vi "MacroGen_MD_old.vi"() -> ()   [LabVIEW 2012]
uses:
  Custom Controls and Typedefs/Available Operations Tree.ctl
  Custom Controls and Typedefs/Edit Button.ctl
  Custom Controls and Typedefs/Delete Button.ctl
  Custom Controls and Typedefs/Macro_MD_UI Control Refnums.ctl
  SubVIs/FormatTree&TableStyle_Commands.ctl
  SubVIs/FGV_MacroGen_Commands.ctl
  Custom Controls and Typedefs/Macro_CommandStruct.ctl
  Custom Controls and Typedefs/Macro_Action_List.ctl
  Custom Controls and Typedefs/Macro_ArgumentStruct.ctl
  CommonResource VIs/FormatTableStyle_Commands.ctl
  <vilib>/Utility/file.llb/Write To Spreadsheet File (string).vi
panel:
  in  "MacroTreeOperation":T3
  in  "File Operation Cluster":cluster{"Load Macro":bool, "SaveAs":bool}
  in  "Table Navigation Cluster":T4
  in  "Parameters":string[][](table)
  in  "Execute Macro":bool
  in  "Add":bool
  in  "Available Actions":T5
  in  "stop":bool
  in  "Macro":string(tree)
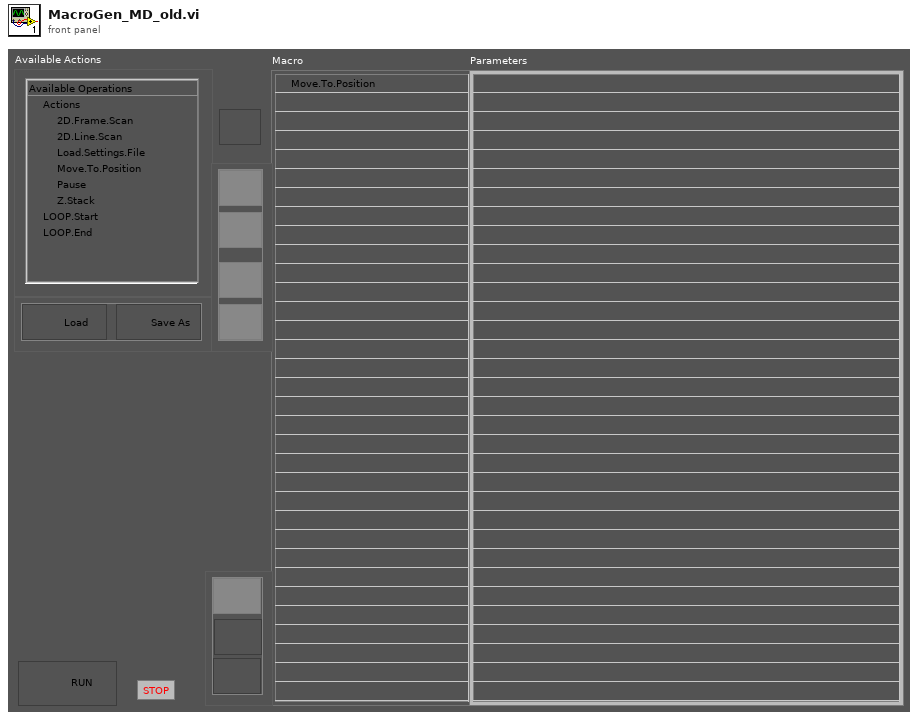
[diagram p1: front panel]
types:
  T1 = typedef "Edit Button.ctl" = bool
  T2 = typedef "Delete Button.ctl" = bool
  T3 = cluster{"Save Button":bool, "Edit Button":T1, "Delete Button":T2}
  T4 = cluster{"Table Index Up":bool, "Table Index Up-End":bool, "Table Index Down":bool, "Table Index Down-End":bool}
  T5 = typedef "Available Operations Tree.ctl" = string
  T6 = typedef "Macro_MD_UI Control Refnums.ctl" = cluster{"Available Operations":refnum<vi>, "Created Macro":refnum<vi>, "Indent Item":refnum<vi>, "Add Selected to Macro":refnum<vi>, "Outdent Item":refnum<vi>, "Number of Iterations":refnum<vi>, "Seconds to Wait":refnum<vi>, "Load Macro":refnum<vi>, "Save Macro":refnum<vi>, "Select File to Load":refnum<vi>, "Params Table":refnum<vi>, "Delete":refnum<vi>, "Edit Button":refnum<vi>, "Execute Macro":refnum<vi>}
  T7 = typedef "FGV_MacroGen_Commands.ctl" = enum16{"Initialize", "Get Array", "Load from file", "Insert Item", "Insert at End", "Edit Item", "Delete Item", "Move Items", "Save", "SaveAs"}
  T8 = typedef "FormatTree&TableStyle_Commands.ctl" = enum16{"Colour Row", "Uncolour Row", "Bold Row", "Unbold Row", "Clear", "UpdateVisibleRows"}
  T9 = typedef "Macro_CommandStruct.ctl" = cluster{"Action":T10, "Arguments":T11[]}
  T10 = typedef "Macro_Action_List.ctl" = enum16{"Unknown", "2D.Frame.Scan", "2D.Line.Scan", "Load.Settings.File", "Move.To.Position", "Pause", "Z.Stack", "LOOP.Start", "LOOP.End"}
  T11 = typedef "Macro_ArgumentStruct.ctl" = cluster{"ArgumentName":string, "DataType":enum16{"Numeric", "String"}, "Value":variant}
  T12 = typedef "FormatTableStyle_Commands.ctl" = enum16{"Colour Row", "Uncolour Row", "Bold Row", "Clear table", "UpdateVisibleRows"}
  T13 = cluster{"data name":string, "drag data":variant}[]
  T14 = typedef "LVPoint32TypeDef.ctl" = cluster{"Horizontal":i32, "Vertical":i32}
  T15 = typedef "LVRowAndColumnTypeDef.ctl" = cluster{"Row":i32, "Column":i32}
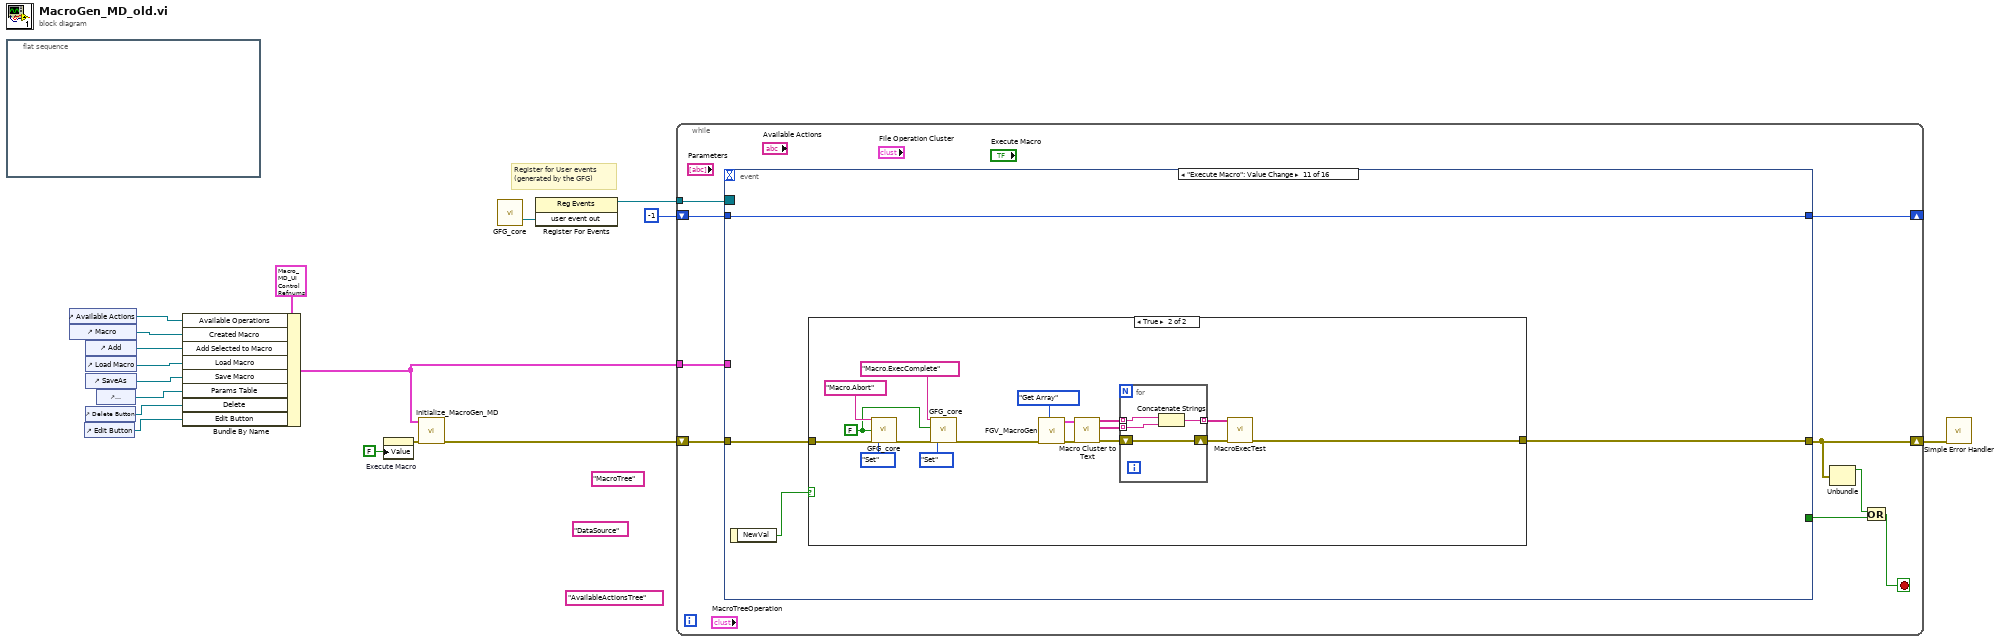
[diagram p0: block diagram]
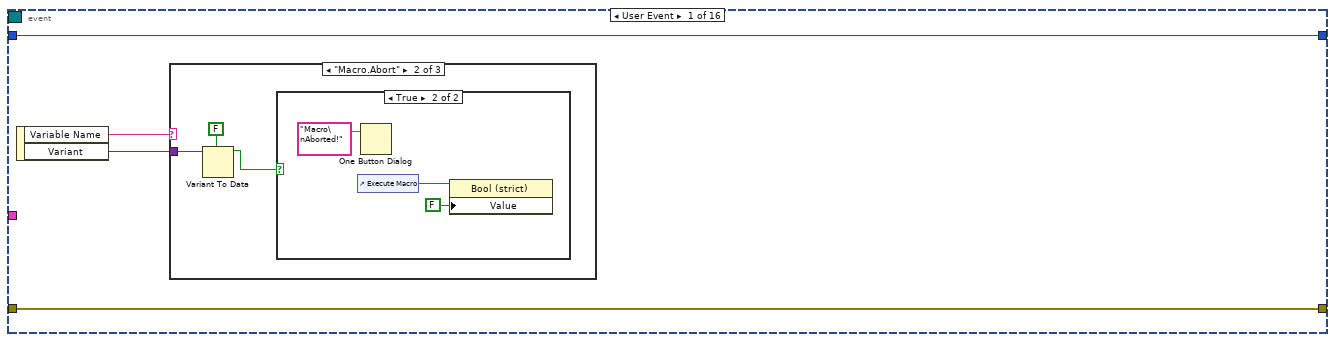
[diagram p2: hidden frame]
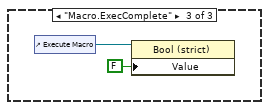
[diagram p5: hidden frame]
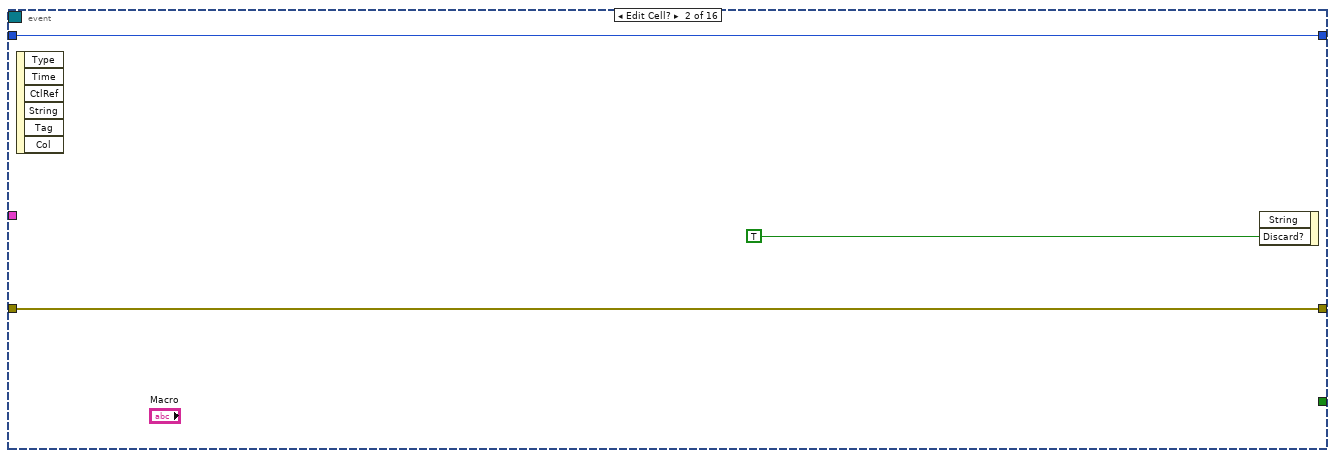
[diagram p6: hidden frame]
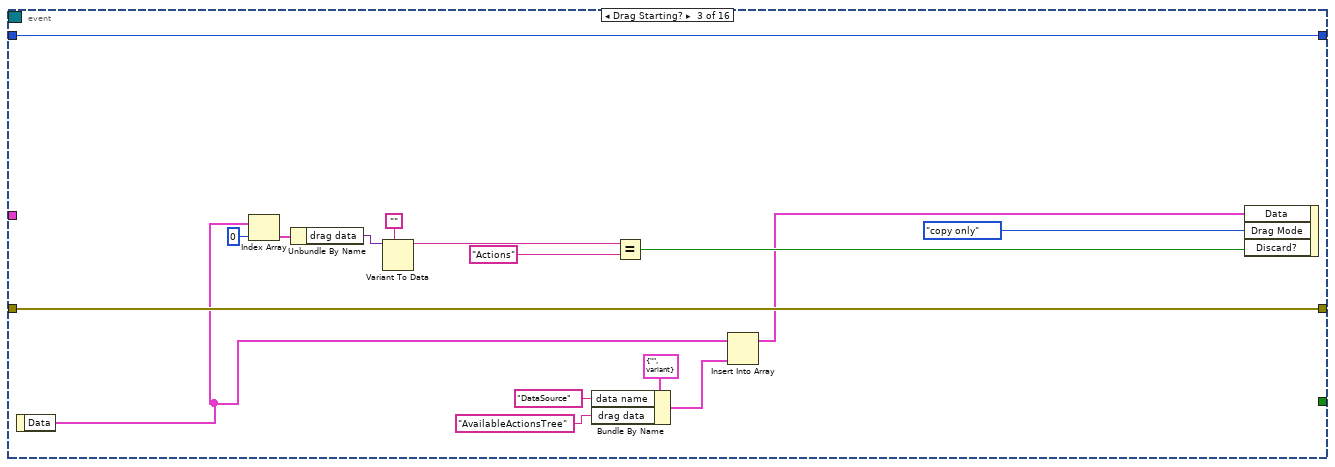
[diagram p7: hidden frame]
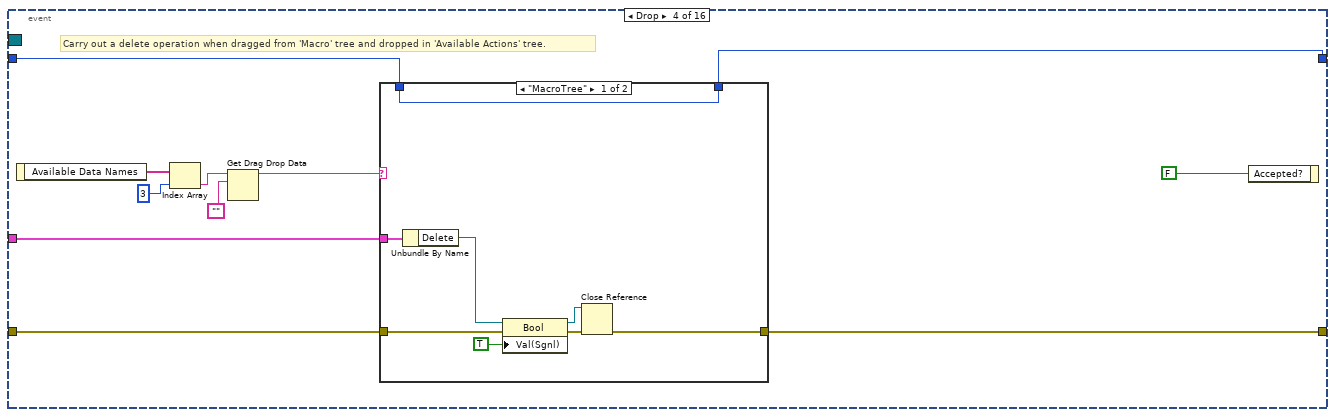
[diagram p8: hidden frame]
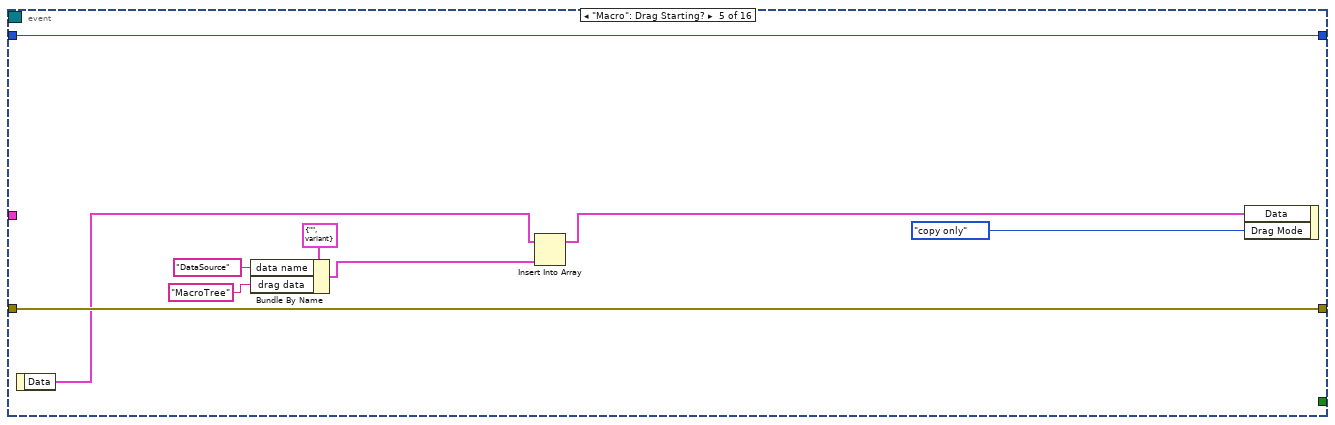
[diagram p10: hidden frame]
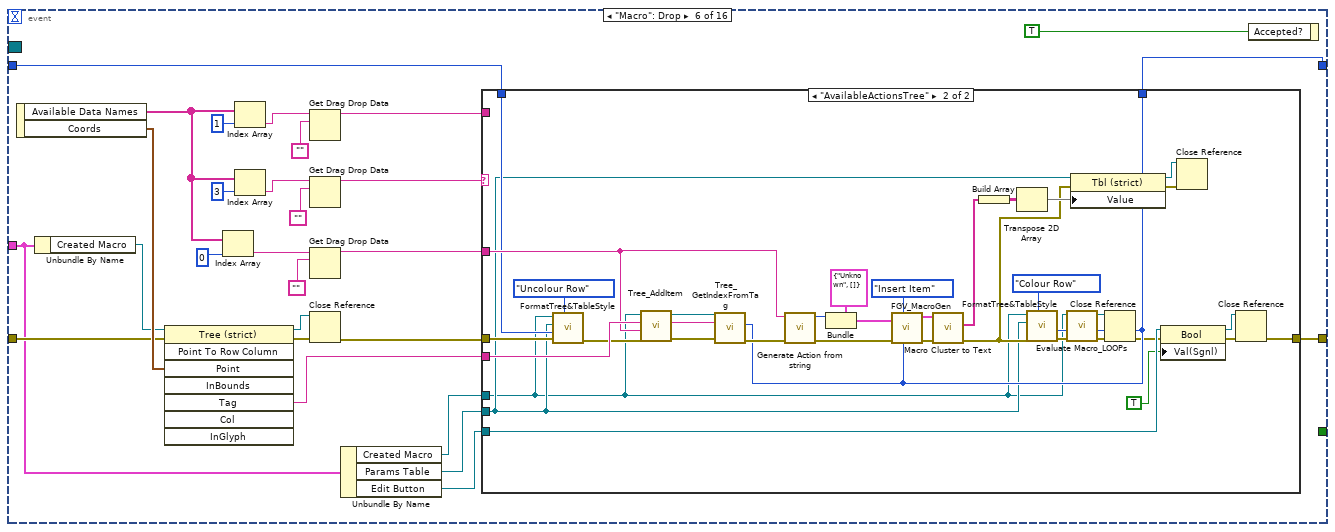
[diagram p11: hidden frame]
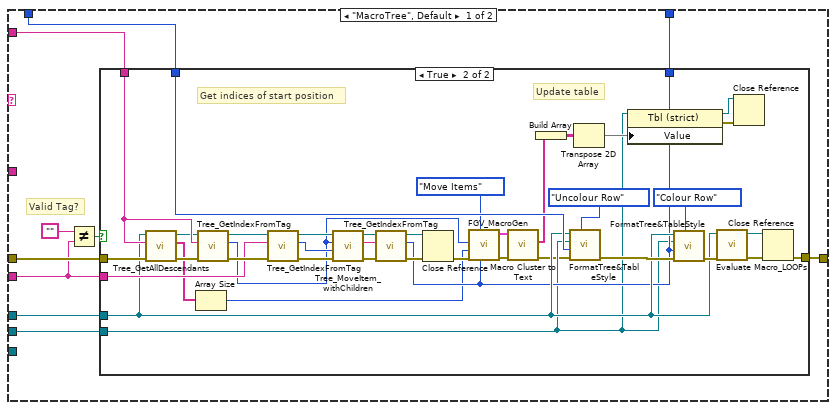
[diagram p12: hidden frame]
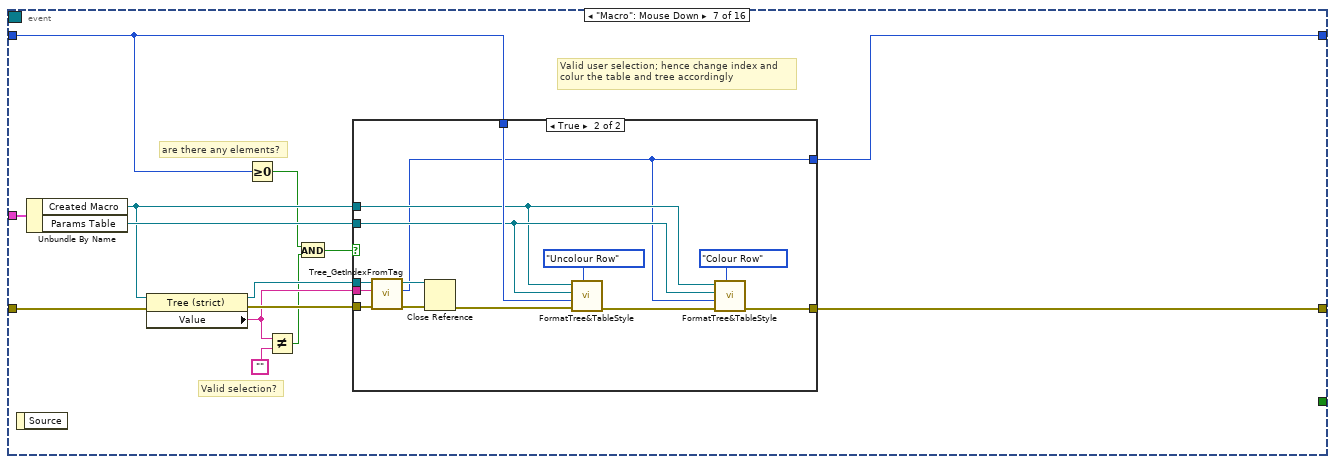
[diagram p14: hidden frame]
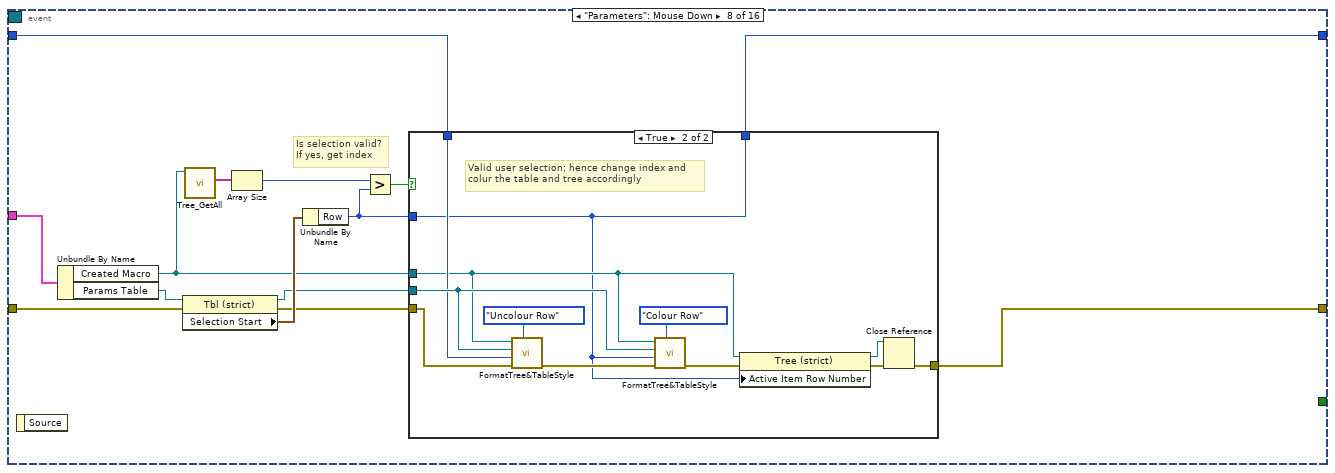
[diagram p16: hidden frame]
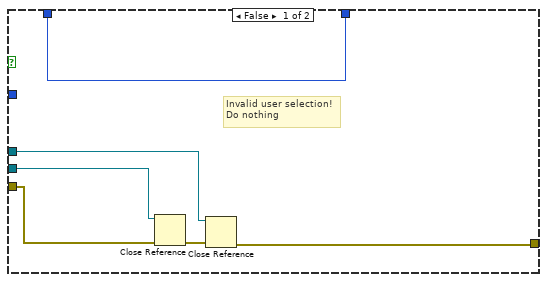
[diagram p17: hidden frame]
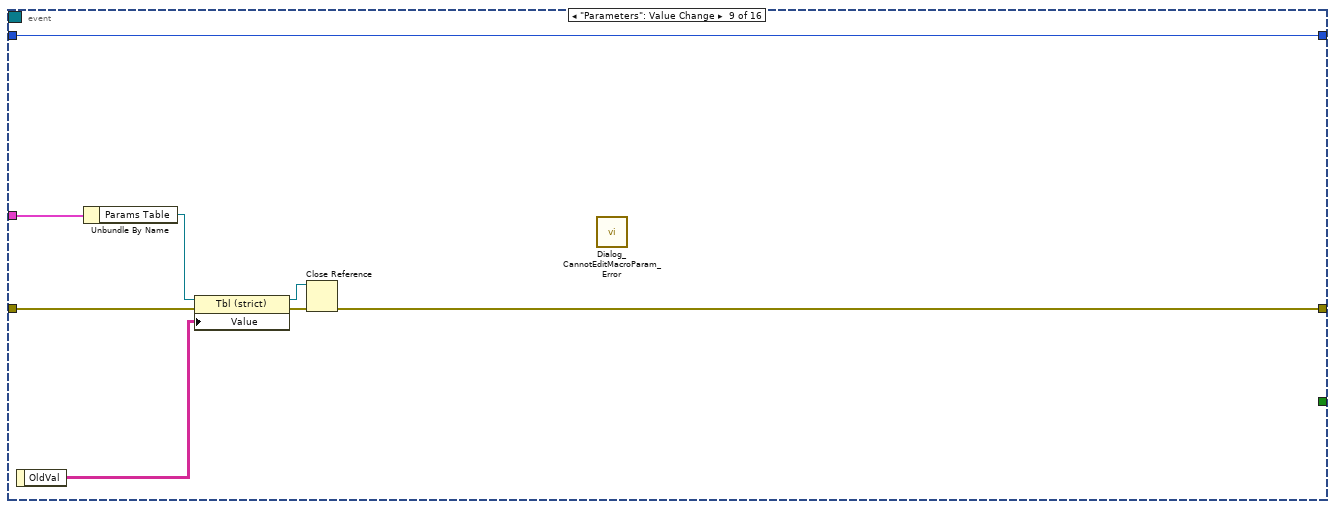
[diagram p18: hidden frame]
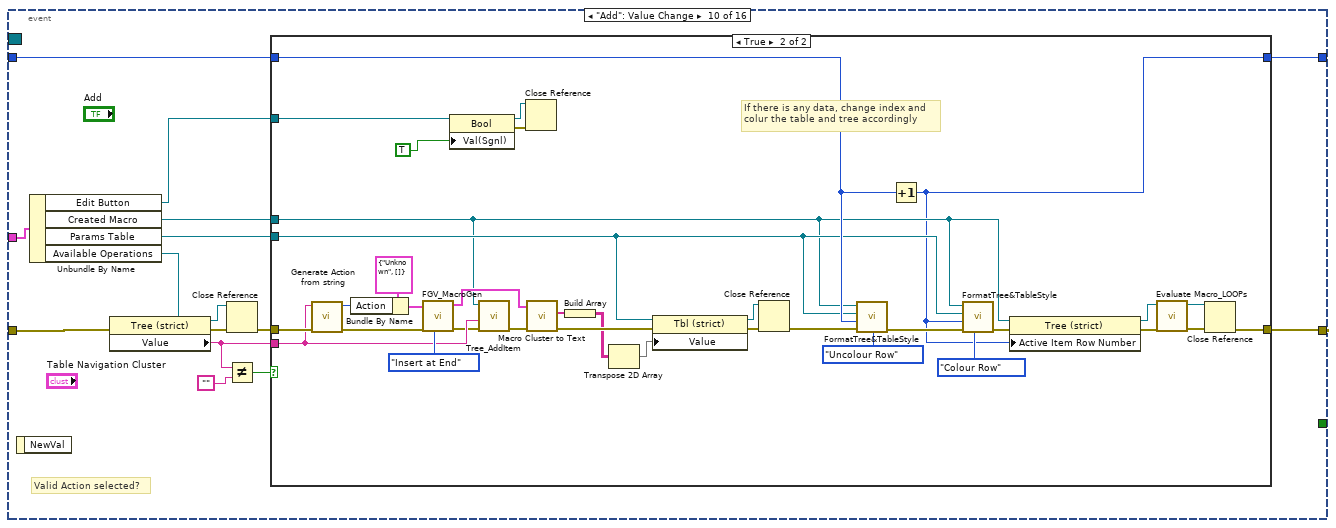
[diagram p19: hidden frame]
diagram:
  (unwired) "MacroTree" ("data name")
  (unwired) "DataSource" ("data name")
  (unwired) "AvailableActionsTree" ("data name")
  # "Register for User events\n(generated by the GFG)"
  n1 = flat-sequence {
    frame #0 {
    }
  }
  n2 = control-ref of="Available Actions"() -> (w7:refnum<vi>)
  n3 = control-ref of="Macro"() -> (w8:refnum<vi>)
  n4 = control-ref of="Edit Button"() -> (w1:refnum<vi>)
  n5 = control-ref of="Delete Button"() -> (w2:refnum<vi>)
  n6 = control-ref of="Add"() -> (w15:refnum<vi>)
  n7 = control-ref of="Load Macro"() -> (w14:refnum<vi>)
  n8 = control-ref of="SaveAs"() -> (w13:refnum<vi>)
  n9 = control-ref of="Parameters"() -> (w9:refnum<vi>)
  n10 = Bundle By Name(cluster=T6 {"Available Operations"=refnum, "Created Macro"=refnum, "Indent Item"=refnum, "Add Selected to Macro"=refnum, "Outdent Item"=refnum, "Number of Iterations"=refnum, "Seconds to Wait"=refnum, "Load Macro"=refnum, "Save Macro"=refnum, "Select File to Load"=refnum, "Params Table"=refnum, "Delete"=refnum, "Edit Button"=refnum, "Execute Macro"=refnum} ("UI control refnums"), "Available Operations"=w7, "Created Macro"=w8, "Add Selected to Macro"=w15, "Load Macro"=w14, "Save Macro"=w13, "Params Table"=w9, "Delete"=w2, "Edit Button"=w1) -> (w11:T6)
  n11 = property on="Execute Macro" class="Bool (strict)"("Value"=FALSE ("Execute Macro")) -> (error out=w3:errorcluster)  [unwired: 2 in, 1 out]
  n12 = call "Initialize_MacroGen_MD.vi"("Error In"=w3, "UI control refnums"=w11) -> ("Error Out"=w10:errorcluster)  [unwired: 9 in]
  n13 = call "GFG_core.vi"() -> ("user event out"=w6:refnum<user-event>)  [unwired: 13 in, 6 out]
  n14 = register-events(w6) -> (reference out=w5:refnum<event-registration>)  [unwired: 2 in, 1 out]
  n15 = while {
    tunnel: w11 -> [w26]
    shift-right: [w22] -> w16
    shift-left: w10 -> [w25]
    shift-right: [w24] -> _
    shift-left: -1 ("Index") -> [w23]
    tunnel: w5 -> [w18]
    stop <- w19 stop-if-true
    n16 = event shown="[10] \"Execute Macro\": Value Change" {
      selector: w18 -> [_ _ _ _ _ _ _ _ _ _ _ _ _ _ _ _]
      dyn-events: _ -> [_ _ _ _ _ _ _ _ _ _ _ _ _ _ _ _]
      timeout: _ -> [_ _ _ _ _ _ _ _ _ _ _ _ _ _ _ _]
      tunnel: [_ _ _ _ _ _ _ _ _ _ _ _ _ _ _ "stop"] -> w21
      tunnel: w26 -> [_ _ _ w59 _ w95 w216 w246 w270 w287 _ w368 _ w415 w463 _]
      tunnel: w25 -> [w30 w40 w57 w58 w87 w108 w211 w239 w271 w281 w325 w354 w400 w409 w453 w501]
      tunnel: [w30 w40 w57 w66 w87 w105 w214 w235 w265 w285 w326 w366 w399 w416 w462 w501] -> w22
      tunnel: [w29 w39 w56 w67 w86 w107 w209 w241 w272 w286 w327 w369 w404 w411 w454 w500] -> w24
      tunnel: w23 -> [w29 w39 w56 w61 w86 w96 w206 w242 w272 w284 w327 w370 w404 w412 w454 w500]
      event User Event {
        n17 = event-data() -> ("Variable Name"=w28:string, "Variant"=w27:variant)  [unwired: 1 in]
        n18 = case shown="\"Macro.Abort\"" w28 {
          tunnel: w27 -> [_ w33 _]
          frame Default {
          }
          frame "Macro.Abort" {
            n19 = Variant To Data(type=FALSE ("Value"), Variant=w33) -> (data=w31:bool)  [unwired: 1 in, 1 out]
            n20 = case shown="True" w31 {
              frame False {
              }
              frame True {
                n21 = control-ref of="Execute Macro"() -> (w36:refnum<vi>)
                n22 = One Button Dialog(message="Macro\nAborted!") -> ()  [unwired: 1 in, 1 out]
                n23 = property class="Bool (strict)"(reference=w36, "Value"=FALSE) -> ()  [unwired: 1 in, 2 out]
              }
            }
          }
          frame "Macro.ExecComplete" {
            n24 = control-ref of="Execute Macro"() -> (w38:refnum<vi>)
            n25 = property class="Bool (strict)"(reference=w38, "Value"=FALSE) -> ()  [unwired: 1 in, 2 out]
          }
        }
      }
      event Edit Cell? {
        n26 = event-data() -> ()  [unwired: 1 in, 6 out]
        n27 = event-data("Discard?"=TRUE) -> ()  [unwired: 2 in, 1 out]
      }
      event Drag Starting? {
        n28 = event-data() -> ("Data"=w43:T13)  [unwired: 1 in]
        n29 = Index Array(array=w43, index=0) -> (element=w54:cluster{"data name":string, "drag data":variant})
        n30 = Unbundle By Name(w54) -> ("drag data"=w53:variant)
        n31 = Variant To Data(type="", Variant=w53) -> (data=w51:string)  [unwired: 1 in, 1 out]
        n32 = Bundle By Name(cluster=cluster{"data name":string, "drag data":variant} {"data name"="", "drag data"=variant} ("element"), "data name"="DataSource", "drag data"="AvailableActionsTree" ("data name")) -> (w44:cluster{"data name":string, "drag data":variant})
        n33 = Equal?(x=w51, y="Actions") -> (x = y?=w49:bool)
        n34 = Insert Into Array(array=w43, new element=w44) -> (w42:T13)  [unwired: 1 in]
        n35 = event-data("Data"=w42, "Drag Mode"=enum32{"copy or move", "copy only", "move only"}."copy only", "Discard?"=w49) -> ()  [unwired: 1 in, 1 out]
      }
      event Drop {
        # "Carry out a delete operation when dragged from 'Macro' tree and dropped in 'Available Actions' tree."
        n36 = event-data() -> ("Available Data Names"=w60:string[])  [unwired: 1 in]
        n37 = Index Array(array=w60, index=3) -> (element=w63:string)
        n38 = Get Drag Drop Data(8:"", 9:w63) -> (3:w62:string)  [unwired: 1 in, 1 out]
        n39 = case shown="\"MacroTree\"" w62 {
          tunnel: [w76 w78] -> w67
          tunnel: w58 -> [w73 w77]
          tunnel: [w69 w77] -> w66
          tunnel: w61 -> [w76 w78]
          tunnel: w59 -> [w75 _]
          frame "MacroTree" {
            n40 = Unbundle By Name(w75) -> ("Delete"=w74:refnum<vi>)
            n41 = property class="Bool"(reference=w74, error in=w73, "Val(Sgnl)"=TRUE) -> (reference out=w70:refnum<vi>, error out=w71:errorcluster)
            n42 = Close Reference(reference=w70, error in (no error)=w71) -> (error out=w69:errorcluster)
          }
          frame Default {
          }
        }
        n43 = event-data("Accepted?"=FALSE) -> ()  [unwired: 1 in, 1 out]
      }
      event "Macro": Drag Starting? {
        n44 = event-data() -> ("Data"=w84:T13)  [unwired: 1 in]
        n45 = Bundle By Name(cluster=cluster{"data name":string, "drag data":variant} {"data name"="", "drag data"=variant} ("element"), "data name"="DataSource", "drag data"="MacroTree" ("data name")) -> (w79:cluster{"data name":string, "drag data":variant})
        n46 = Insert Into Array(array=w84, new element=w79) -> (w83:T13)  [unwired: 1 in]
        n47 = event-data("Data"=w83, "Drag Mode"=enum32{"copy or move", "copy only", "move only"}."copy only") -> ()  [unwired: 1 in, 1 out]
      }
      event "Macro": Drop {
        n48 = event-data() -> ("Available Data Names"=w89:string[], "Coords"=w111:T14)  [unwired: 1 in]
        n49 = Unbundle By Name(w95) -> ("Created Macro"=w110:refnum<vi>)
        n50 = invoke class="Tree (strict)" method="Point To Row Column"(reference=w110, error in=w108, "Point"=w111) -> (reference out=w91:refnum<vi>, error out=w92:errorcluster, "Tag"=w109:string)  [unwired: 5 in, 5 out]
        n51 = Index Array(array=w89, index=0) -> (element=w113:string)
        n52 = Index Array(array=w89, index=1) -> (element=w100:string)
        n53 = Index Array(array=w89, index=3) -> (element=w102:string)
        n54 = Get Drag Drop Data(8:"", 9:w100) -> (3:w97:string)  [unwired: 1 in, 1 out]
        n55 = Get Drag Drop Data(8:"", 9:w102) -> (3:w101:string)  [unwired: 1 in, 1 out]
        n56 = Get Drag Drop Data(8:"", 9:w113) -> (3:w106:string)  [unwired: 1 in, 1 out]
        n57 = Close Reference(reference=w91, error in (no error)=w92) -> (error out=w90:errorcluster)
        n58 = Unbundle By Name(w95) -> ("Created Macro"=w94:refnum<vi>, "Params Table"=w93:refnum<vi>, "Edit Button"=w88:refnum<vi>)
        n59 = case shown="\"AvailableActionsTree\"" w101 {
          tunnel: w109 -> [w117 w202]
          tunnel: [w122 w194] -> w107
          tunnel: w90 -> [w125 w193]
          tunnel: w106 -> [_ w200]
          tunnel: [w120 w167] -> w105
          tunnel: w97 -> [w124 _]
          tunnel: w96 -> [w123 w195]
          tunnel: w94 -> [w119 w181]
          tunnel: w93 -> [w121 w183]
          tunnel: w88 -> [_ w172]
          frame "MacroTree", Default {
            # "Valid Tag?"
            n60 = Not Equal?(x="", y=w117) -> (x != y?=w118:bool)
            n61 = case shown="True" w118 {
              tunnel: w125 -> [w126 w146]
              tunnel: w117 -> [_ w162]
              tunnel: w124 -> [_ w147]
              tunnel: w123 -> [w127 w158]
              tunnel: [w127 w139] -> w122
              tunnel: w121 -> [_ w133]
              tunnel: [w126 w154] -> w120
              tunnel: w119 -> [_ w144]
              frame False {
              }
              frame True {
                # "Update table"
                # "Get indices of start position"
                n62 = call "Tree_GetAllDescendants.vi"("Error In"=w146, "Tag"=w147, "Tree Refnum IN"=w144) -> ("Error Out"=w145:errorcluster, "All Descendants"=w142:string[], "Tree Refnum OUT"=w143:refnum<vi>)  [unwired: 6 in]
                n63 = Array Size(array=w142) -> (size(s)=w137:i32)
                n64 = call "Tree_GetIndexFromTag.vi"("Error In"=w145, "Tag IN"=w147, "Tree Refnum IN"=w143) -> ("Error Out"=w165:errorcluster, "Index OUT"=w138:i32, "Tree Refnum OUT"=w166:refnum<vi>)  [unwired: 6 in]
                n65 = call "Tree_GetIndexFromTag.vi"("Error In"=w165, "Tag IN"=w162, "Tree Refnum IN"=w166) -> ("Error Out"=w164:errorcluster, "Index OUT"=w157:i32, "Tree Refnum OUT"=w163:refnum<vi>)  [unwired: 6 in]
                n66 = call "Tree_MoveItem_withChildren.vi"("Error In"=w164, "End Index"=w157, "Start Index"=w138, "Tree Refnum IN"=w163) -> ("Error Out"=w151:errorcluster, "Moved Tag"=w149:string, "Tree Refnum OUT"=w150:refnum<vi>)  [unwired: 5 in]
                n67 = call "Tree_GetIndexFromTag.vi"("Error In"=w151, "Tag IN"=w149, "Tree Refnum IN"=w150) -> ("Error Out"=w152:errorcluster, "Index OUT"=w139:i32, "Tree Refnum OUT"=w148:refnum<vi>)  [unwired: 6 in]
                n68 = Close Reference(reference=w148, error in (no error)=w152) -> (error out=w140:errorcluster)
                n69 = call "FGV_MacroGen.vi"("Final Index"=w139, "MacroFGV_Commands"=FGV_MacroGen_Commands."Move Items", "Error In"=w140, "Length"=w137, "Start Index"=w138) -> ("Error Out"=w131:errorcluster, "Macro Cluster Array"=w132:T9[])  [unwired: 4 in, 1 out]
                n70 = call "Macro Cluster to Text.vi"("Error In"=w131, "Macro Cluster Array IN"=w132) -> ("Error Out"=w130:errorcluster, "Argument List (Txt)"=w129:string[])  [unwired: 7 in, 1 out]
                n71 = Build Array(w129) -> (w135:string[][])
                n72 = call "FormatTree&TableStyle.vi"("Format Command"=FormatTree&TableStyle_Commands."Uncolour Row", "Error In"=w130, "Row Index"=w158, "Tbl Refnum"=w133, "Tree Refnum"=w144) -> ("Error Out"=w159:errorcluster)  [unwired: 6 in]
                n73 = Transpose 2D Array(2D array=w135) -> (transposed array=w134:string[][])
                n74 = property class="Tbl (strict)"(reference=w133, "Value"=w134) -> (reference out=w128:refnum<vi>, error out=w136:errorcluster)  [unwired: 1 in]
                n75 = call "FormatTree&TableStyle.vi"("Format Command"=FormatTree&TableStyle_Commands."Colour Row", "Error In"=w159, "Row Index"=w139, "Tbl Refnum"=w133, "Tree Refnum"=w144) -> ("Error Out"=w155:errorcluster)  [unwired: 6 in]
                n76 = call "Evaluate Macro_LOOPs.vi"("Error In"=w155, "Tree Refnum IN"=w144) -> ("Error Out"=w156:errorcluster, "Tree Refnum OUT"=w153:refnum<vi>)  [unwired: 7 in, 1 out]
                n77 = Close Reference(reference=w128, error in (no error)=w136) -> ()  [unwired: 1 out]
                n78 = Close Reference(reference=w153, error in (no error)=w156) -> (error out=w154:errorcluster)
              }
            }
          }
          frame "AvailableActionsTree" {
            n79 = call "FormatTree&TableStyle.vi"("Format Command"=FormatTree&TableStyle_Commands."Uncolour Row", "Error In"=w193, "Row Index"=w195, "Tbl Refnum"=w183, "Tree Refnum"=w181) -> ("Error Out"=w192:errorcluster)  [unwired: 6 in]
            n80 = call "Tree_AddItem.vi"("Error In"=w192, "NEW String"=w200, "Tag at add position"=w202, "Tree Refnum"=w181) -> ("Error Out"=w178:errorcluster, "Added Item Tag"=w176:string, "Tree Refnum OUT"=w177:refnum<vi>)  [unwired: 5 in]
            n81 = call "Tree_GetIndexFromTag.vi"("Error In"=w178, "Tag IN"=w176, "Tree Refnum IN"=w177) -> ("Error Out"=w198:errorcluster, "Index OUT"=w194:i32)  [unwired: 6 in, 1 out]
            n82 = call "Generate Action from string.vi"("Error In"=w198, "Command Text"=w200) -> ("Error Out"=w199:errorcluster, "Action"=w174:T10)  [unwired: 8 in]
            n83 = Bundle(cluster=T9 {"Action"=enum."Unknown", "Arguments"=[]} ("Macro Commands"), "Action"=w174) -> (w173:T9)  [unwired: 1 in]
            n84 = call "FGV_MacroGen.vi"("Final Index"=w194, "MacroFGV_Commands"=FGV_MacroGen_Commands."Insert Item", "Error In"=w199, "Macro Command IN"=w173) -> ("Error Out"=w185:errorcluster, "Macro Cluster Array"=w186:T9[])  [unwired: 5 in, 1 out]
            n85 = call "Macro Cluster to Text.vi"("Error In"=w185, "Macro Cluster Array IN"=w186) -> ("Error Out"=w184:errorcluster, "Argument List (Txt)"=w191:string[])  [unwired: 7 in, 1 out]
            n86 = Build Array(w191) -> (w188:string[][])
            n87 = Transpose 2D Array(2D array=w188) -> (transposed array=w187:string[][])
            n88 = call "FormatTree&TableStyle.vi"("Format Command"=FormatTree&TableStyle_Commands."Colour Row", "Error In"=w184, "Row Index"=w194, "Tbl Refnum"=w183, "Tree Refnum"=w181) -> ("Error Out"=w182:errorcluster)  [unwired: 6 in]
            n89 = call "Evaluate Macro_LOOPs.vi"("Error In"=w182, "Tree Refnum IN"=w181) -> ("Error Out"=w180:errorcluster, "Tree Refnum OUT"=w179:refnum<vi>)  [unwired: 7 in, 1 out]
            n90 = property class="Tbl (strict)"(reference=w183, error in=w184, "Value"=w187) -> (reference out=w189:refnum<vi>, error out=w190:errorcluster)
            n91 = Close Reference(reference=w179, error in (no error)=w180) -> (error out=w171:errorcluster)
            n92 = property class="Bool"(reference=w172, error in=w171, "Val(Sgnl)"=TRUE) -> (reference out=w168:refnum<vi>, error out=w169:errorcluster)
            n93 = Close Reference(reference=w189, error in (no error)=w190) -> ()  [unwired: 1 out]
            n94 = Close Reference(reference=w168, error in (no error)=w169) -> (error out=w167:errorcluster)
          }
        }
        n95 = event-data("Accepted?"=TRUE) -> ()  [unwired: 1 in, 1 out]
      }
      event "Macro": Mouse Down {
        # "are there any elements?"
        # "Valid selection?"
        # "Valid user selection; hence change index and\ncolur the table and tree accordingly"
        n96 = event-data() -> ()  [unwired: 1 in, 1 out]
        n97 = Unbundle By Name(w216) -> ("Created Macro"=w212:refnum<vi>, "Params Table"=w215:refnum<vi>)
        n98 = property class="Tree (strict)"(reference=w212, error in=w211) -> (reference out=w210:refnum<vi>, error out=w213:errorcluster, "Value"=w208:string)
        n99 = Greater Or Equal To 0?(x=w206) -> (x >= 0?=w205:bool)
        n100 = Not Equal?(x=w208, y="") -> (x != y?=w204:bool)
        n101 = And(x=w205, y=w204) -> (x .and. y?=w203:bool)
        n102 = case shown="True" w203 {
          tunnel: w206 -> [w218 w232]
          tunnel: w215 -> [_ w231]
          tunnel: [w217 w230] -> w214
          tunnel: w213 -> [w217 w219]
          tunnel: w212 -> [_ w229]
          tunnel: w210 -> [_ w220]
          tunnel: w208 -> [_ w221]
          tunnel: [w218 w225] -> w209
          frame False {
          }
          frame True {
            n103 = call "Tree_GetIndexFromTag.vi"("Error In"=w219, "Tag IN"=w221, "Tree Refnum IN"=w220) -> ("Error Out"=w227:errorcluster, "Index OUT"=w225:i32, "Tree Refnum OUT"=w226:refnum<vi>)  [unwired: 6 in]
            n104 = Close Reference(reference=w226, error in (no error)=w227) -> (error out=w228:errorcluster)
            n105 = call "FormatTree&TableStyle.vi"("Format Command"=FormatTree&TableStyle_Commands."Uncolour Row", "Error In"=w228, "Row Index"=w232, "Tbl Refnum"=w231, "Tree Refnum"=w229) -> ("Error Out"=w222:errorcluster)  [unwired: 6 in]
            n106 = call "FormatTree&TableStyle.vi"("Format Command"=FormatTree&TableStyle_Commands."Colour Row", "Error In"=w222, "Row Index"=w225, "Tbl Refnum"=w231, "Tree Refnum"=w229) -> ("Error Out"=w230:errorcluster)  [unwired: 6 in]
          }
        }
      }
      event "Parameters": Mouse Down {
        # "Is selection valid?\nIf yes, get index"
        n107 = event-data() -> ()  [unwired: 1 in, 1 out]
        n108 = Unbundle By Name(w246) -> ("Created Macro"=w233:refnum<vi>, "Params Table"=w240:refnum<vi>)
        n109 = property class="Tbl (strict)"(reference=w240, error in=w239) -> (reference out=w237:refnum<vi>, error out=w236:errorcluster, "Selection Start"=w245:T15)
        n110 = call "Tree_GetAll.vi"("Tree Refnum IN"=w233) -> ("Tags"=w234:string[])  [unwired: 7 in, 3 out]
        n111 = Array Size(array=w234) -> (size(s)=w244:i32)
        n112 = Unbundle By Name(w245) -> ("Row"=w238:i32)
        n113 = Greater?(x=w244, y=w238) -> (0:w243:bool)
        n114 = case shown="True" w243 {
          tunnel: w242 -> [w252 w259]
          tunnel: [w252 w256] -> w241
          tunnel: w237 -> [w248 w260]
          tunnel: w233 -> [w247 w258]
          tunnel: w238 -> [_ w256]
          tunnel: w236 -> [w251 w262]
          tunnel: [w249 w253] -> w235
          frame False {
            # "Invalid user selection!\nDo nothing"
            n115 = Close Reference(reference=w248, error in (no error)=w251) -> (error out=w250:errorcluster)
            n116 = Close Reference(reference=w247, error in (no error)=w250) -> (error out=w249:errorcluster)
          }
          frame True {
            # "Valid user selection; hence change index and\ncolur the table and tree accordingly"
            n117 = call "FormatTree&TableStyle.vi"("Format Command"=FormatTree&TableStyle_Commands."Uncolour Row", "Error In"=w262, "Row Index"=w259, "Tbl Refnum"=w260, "Tree Refnum"=w258) -> ("Error Out"=w261:errorcluster)  [unwired: 6 in]
            n118 = call "FormatTree&TableStyle.vi"("Format Command"=FormatTree&TableStyle_Commands."Colour Row", "Error In"=w261, "Row Index"=w256, "Tbl Refnum"=w260, "Tree Refnum"=w258) -> ("Error Out"=w257:errorcluster)  [unwired: 6 in]
            n119 = property class="Tree (strict)"(reference=w258, error in=w257, "Active Item Row Number"=w256) -> (reference out=w254:refnum<vi>, error out=w255:errorcluster)
            n120 = Close Reference(reference=w254, error in (no error)=w255) -> (error out=w253:errorcluster)
          }
        }
      }
      event "Parameters": Value Change {
        n121 = event-data() -> ("OldVal"=w268:string[][])  [unwired: 1 in]
        n122 = Unbundle By Name(w270) -> ("Params Table"=w269:refnum<vi>)
        n123 = property class="Tbl (strict)"(reference=w269, error in=w271, "Value"=w268) -> (reference out=w266:refnum<vi>, error out=w267:errorcluster)
        n124 = Close Reference(reference=w266, error in (no error)=w267) -> (error out=w265:errorcluster)
        n125 = call "Dialog_CannotEditMacroParam_Error.vi"() -> ()  [unwired: 12 in]
      }
      event "Add": Value Change {
        # "Valid Action selected?"
        n126 = event-data() -> ()  [unwired: 1 in, 1 out]
        n127 = Unbundle By Name(w287) -> ("Edit Button"=w273:refnum<vi>, "Created Macro"=w274:refnum<vi>, "Params Table"=w283:refnum<vi>, "Available Operations"=w282:refnum<vi>)
        n128 = property class="Tree (strict)"(reference=w282, error in=w281) -> (reference out=w277:refnum<vi>, error out=w278:errorcluster, "Value"=w275:string)
        n129 = Close Reference(reference=w277, error in (no error)=w278) -> (error out=w276:errorcluster)
        n130 = Not Equal?(x=w275, y="") -> (x != y?=w279:bool)
        n131 = case shown="True" w279 {
          tunnel: [w289 w301] -> w286
          tunnel: [w288 w302] -> w285
          tunnel: w284 -> [w289 w323]
          tunnel: w283 -> [_ w315]
          tunnel: w276 -> [w288 w322]
          tunnel: w275 -> [_ w319]
          tunnel: w274 -> [_ w304]
          tunnel: w273 -> [_ w293]
          frame False {
          }
          frame True {
            # "If there is any data, change index and\ncolur the table and tree accordingly"
            n132 = call "Generate Action from string.vi"("Error In"=w322, "Command Text"=w319) -> ("Error Out"=w320:errorcluster, "Action"=w295:T10)  [unwired: 8 in]
            n133 = Bundle By Name(cluster=T9 {"Action"=enum."Unknown", "Arguments"=[]} ("Macro Commands"), "Action"=w295) -> (w294:T9)
            n134 = call "FGV_MacroGen.vi"("MacroFGV_Commands"=FGV_MacroGen_Commands."Insert at End", "Error In"=w320, "Macro Command IN"=w294) -> ("Error Out"=w318:errorcluster, "Macro Cluster Array"=w317:T9[])  [unwired: 6 in, 1 out]
            n135 = property class="Bool"(reference=w293, "Val(Sgnl)"=TRUE) -> (reference out=w290:refnum<vi>, error out=w291:errorcluster)  [unwired: 1 in]
            n136 = call "Tree_AddItem.vi"("Error In"=w318, "NEW String"=w319, "Tree Refnum"=w304) -> ("Error Out"=w316:errorcluster)  [unwired: 6 in, 2 out]
            n137 = Close Reference(reference=w290, error in (no error)=w291) -> ()  [unwired: 1 out]
            n138 = call "Macro Cluster to Text.vi"("Error In"=w316, "Macro Cluster Array IN"=w317) -> ("Error Out"=w313:errorcluster, "Argument List (Txt)"=w314:string[])  [unwired: 7 in, 1 out]
            n139 = Build Array(w314) -> (w306:string[][])
            n140 = Transpose 2D Array(2D array=w306) -> (transposed array=w305:string[][])
            n141 = property class="Tbl (strict)"(reference=w315, error in=w313, "Value"=w305) -> (reference out=w311:refnum<vi>, error out=w312:errorcluster)
            n142 = Close Reference(reference=w311, error in (no error)=w312) -> (error out=w310:errorcluster)
            n143 = call "FormatTree&TableStyle.vi"("Format Command"=FormatTree&TableStyle_Commands."Uncolour Row", "Error In"=w310, "Row Index"=w323, "Tbl Refnum"=w315, "Tree Refnum"=w304) -> ("Error Out"=w307:errorcluster)  [unwired: 6 in]
            n144 = Increment(x=w323) -> (x+1=w301:i32)
            n145 = call "FormatTree&TableStyle.vi"("Format Command"=FormatTree&TableStyle_Commands."Colour Row", "Error In"=w307, "Row Index"=w301, "Tbl Refnum"=w315, "Tree Refnum"=w304) -> ("Error Out"=w303:errorcluster)  [unwired: 6 in]
            n146 = property class="Tree (strict)"(reference=w304, error in=w303, "Active Item Row Number"=w301) -> (reference out=w299:refnum<vi>, error out=w300:errorcluster)
            n147 = call "Evaluate Macro_LOOPs.vi"("Error In"=w300, "Tree Refnum IN"=w299) -> ("Error Out"=w298:errorcluster, "Tree Refnum OUT"=w297:refnum<vi>)  [unwired: 7 in, 1 out]
            n148 = Close Reference(reference=w297, error in (no error)=w298) -> (error out=w302:errorcluster)
          }
        }
      }
      event "Execute Macro": Value Change {
        n149 = event-data() -> ("NewVal"=w324:bool)  [unwired: 1 in]
        n150 = case shown="True" w324 {
          tunnel: [w328 w335] -> w326
          tunnel: w325 -> [w329 w334]
          frame False {
            n151 = call "GFG_core.vi"("Variable Name in"="Macro.Abort", "Variant in"=TRUE, "error in (no error)"=w329, "Action"=enum16{"Init", "Set", "Get", "Clear"}."Set") -> ("error out"=w328:errorcluster)  [unwired: 9 in, 6 out]
          }
          frame True {
            w333 = FALSE
            n152 = call "GFG_core.vi"("Variable Name in"="Macro.Abort", "Variant in"=w333, "error in (no error)"=w334, "Action"=enum16{"Init", "Set", "Get", "Clear"}."Set") -> ("error out"=w338:errorcluster)  [unwired: 9 in, 6 out]
            n153 = call "GFG_core.vi"("Variable Name in"="Macro.ExecComplete", "Variant in"=w333, "error in (no error)"=w338, "Action"=enum16{"Init", "Set", "Get", "Clear"}."Set") -> ("error out"=w346:errorcluster)  [unwired: 9 in, 6 out]
            n154 = call "FGV_MacroGen.vi"("MacroFGV_Commands"=FGV_MacroGen_Commands."Get Array", "Error In"=w346) -> ("Error Out"=w345:errorcluster, "Macro Cluster Array"=w344:T9[])  [unwired: 7 in, 1 out]
            n155 = call "Macro Cluster to Text.vi"("Error In"=w345, "Macro Cluster Array IN"=w344) -> ("Error Out"=w341:errorcluster, "Argument List (Txt)"=w342:string[], "Action List (Txt)"=w343:string[])  [unwired: 7 in]
            n156 = for {
              tunnel: w343 -> [w353] mode=indexing
              tunnel: w342 -> [w352] mode=indexing
              tunnel: [w351] -> w336 mode=indexing
              shift-right: [w350] -> w337
              shift-left: w341 -> [w350]
              n157 = Concatenate Strings(w353, w352) -> (w351:string)
            }
            n158 = call "MacroExecTest.vi"("Error In"=w337, "Macro IN"=w336) -> ("Error Out"=w335:errorcluster)  [unwired: 9 in]
          }
        }
      }
      event "File Operation Cluster.Load Macro": Value Change {
        w369 = 0 ("Index")
        # "Clear tree first"
        # "Reverse array as items are being added to the top level"
        # "New Index"
        n159 = event-data() -> ()  [unwired: 1 in, 1 out]
        n160 = Unbundle By Name(w368) -> ("Created Macro"=w360:refnum<vi>, "Params Table"=w367:refnum<vi>)
        n161 = call "FGV_MacroGen.vi"("MacroFGV_Commands"=FGV_MacroGen_Commands."Load from file", "Error In"=w354) -> ("Error Out"=w372:errorcluster, "Macro Cluster Array"=w371:T9[])  [unwired: 7 in, 1 out]
        n162 = call "Macro Cluster to Text.vi"("Error In"=w372, "Macro Cluster Array IN"=w371) -> ("Error Out"=w385:errorcluster, "Argument List (Txt)"=w386:string[], "Action List (Txt)"=w362:string[])  [unwired: 7 in]
        n163 = Build Array(w386) -> (w379:string[][])
        n164 = Transpose 2D Array(2D array=w379) -> (transposed array=w378:string[][])
        n165 = property class="Tbl (strict)"(reference=w367, error in=w385, "Value"=w378) -> (reference out=w383:refnum<vi>, error out=w384:errorcluster)
        n166 = Close Reference(reference=w383, error in (no error)=w384) -> (error out=w357:errorcluster)
        n167 = invoke class="Tree (strict)" method="Edit Tree Items.Delete"(reference=w360, error in=w357, "tag"="" ("Tag"), "Delete Children"=TRUE ("Delete Children?")) -> (reference out=w355:refnum<vi>, error out=w356:errorcluster)  [unwired: 1 in, 3 out]
        n168 = Reverse 1D Array(array=w362) -> (reversed array=w361:string[])
        n169 = for {
          tunnel: w361 -> [w391] mode=indexing
          shift-right: [w389] -> w365
          shift-left: w356 -> [w390]
          shift-right: [w388] -> w364
          shift-left: w355 -> [w392]
          # "Add items to tree"
          n170 = invoke class="Tree (strict)" method="Edit Tree Items.Add Item"(reference=w392, error in=w390, "Left Cell"=w391) -> (reference out=w388:refnum<vi>, error out=w389:errorcluster)  [unwired: 6 in, 7 out]
        }
        n171 = Close Reference(reference=w364, error in (no error)=w365) -> (error out=w363:errorcluster)
        n172 = call "FormatTree&TableStyle.vi"("Format Command"=FormatTree&TableStyle_Commands."Uncolour Row", "Error In"=w363, "Row Index"=w370, "Tbl Refnum"=w367, "Tree Refnum"=w360) -> ("Error Out"=w380:errorcluster)  [unwired: 6 in]
        n173 = call "FormatTree&TableStyle.vi"("Format Command"=FormatTree&TableStyle_Commands."Colour Row", "Error In"=w380, "Row Index"=w369, "Tbl Refnum"=w367, "Tree Refnum"=w360) -> ("Error Out"=w377:errorcluster)  [unwired: 6 in]
        n174 = property class="Tree (strict)"(reference=w360, error in=w377, "Active Item Row Number"=w369) -> (reference out=w375:refnum<vi>, error out=w376:errorcluster)
        n175 = call "Evaluate Macro_LOOPs.vi"("Error In"=w376, "Tree Refnum IN"=w375) -> ("Error Out"=w374:errorcluster, "Tree Refnum OUT"=w373:refnum<vi>)  [unwired: 7 in, 1 out]
        n176 = Close Reference(reference=w373, error in (no error)=w374) -> (error out=w366:errorcluster)
      }
      event "File Operation Cluster.SaveAs": Value Change {
        n177 = event-data() -> ()  [unwired: 1 in, 1 out]
        n178 = call "FGV_MacroGen.vi"("MacroFGV_Commands"=FGV_MacroGen_Commands."Get Array", "Error In"=w400) -> ("Error Out"=w401:errorcluster, "Macro Cluster Array"=w402:T9[])  [unwired: 7 in, 1 out]
        n179 = call "Macro Cluster to Text.vi"("Error In"=w401, "Macro Cluster Array IN"=w402) -> ("Error Out"=w399:errorcluster, "Argument List (Txt)"=w397:string[], "Action List (Txt)"=w398:string[])  [unwired: 7 in]
        n180 = call "File Dialog"("pattern (all files)"="*.txt") -> ("selected path"=w393:path)  [unwired: 11 in, 3 out]
        n181 = Build Array(w398, w397) -> (w396:string[][])
        n182 = Transpose 2D Array(2D array=w396) -> (transposed array=w395:string[][])
        n183 = call-poly <vilib>:"Write To Spreadsheet File.vi"("2D data"=w395, "file path (dialog if empty)"=w393) -> ()  [unwired: 6 in, 1 out]
      }
      event Value Change {
        n184 = event-data() -> ()  [unwired: 1 in, 4 out]
        n185 = Unbundle By Name(w415) -> ("Created Macro"=w405:refnum<vi>, "Params Table"=w410:refnum<vi>)
        n186 = call "Tree_GetAll.vi"("Error In"=w409, "Tree Refnum IN"=w405) -> ("Error Out"=w408:errorcluster, "Tags"=w407:string[], "Tree Refnum OUT"=w406:refnum<vi>)  [unwired: 6 in, 1 out]
        n187 = Array Size(array=w407) -> (size(s)=w414:i32)
        n188 = Greater Than 0?(x=w414) -> (x > 0?=w413:bool)
        n189 = case shown="True" w413 {
          tunnel: w415 -> [_ _]
          tunnel: w408 -> [w418 w449]
          tunnel: [w418 w427] -> w416
          tunnel: w412 -> [w417 w422]
          tunnel: [w417 w428] -> w411
          tunnel: w406 -> [_ w447]
          tunnel: w410 -> [_ w435]
          frame False {
          }
          frame True {
            n190 = call "FGV_MacroGen.vi"("Final Index"=w422, "MacroFGV_Commands"=FGV_MacroGen_Commands."Delete Item", "Error In"=w449) -> ("Error Out"=w441:errorcluster, "Macro Cluster Array"=w436:T9[])  [unwired: 6 in, 1 out]
            n191 = property class="Tree"(reference=w447, error in=w441, "Active Item Row Number"=w422) -> (reference out=w446:refnum<vi>, error out=w445:errorcluster)
            n192 = call "Macro Cluster to Text.vi"("Macro Cluster Array IN"=w436) -> ("Error Out"=w439:errorcluster, "Argument List (Txt)"=w440:string[])  [unwired: 8 in, 1 out]
            n193 = Build Array(w440) -> (w438:string[][])
            n194 = Transpose 2D Array(2D array=w438) -> (transposed array=w437:string[][])
            n195 = property class="Tree"(reference=w446, error in=w445) -> (reference out=w443:refnum<vi>, error out=w442:errorcluster, "Active Item Tag"=w444:string)
            n196 = property class="Tbl (strict)"(reference=w435, error in=w439, "Value"=w437) -> (reference out=w424:refnum<vi>)  [unwired: 1 out]
            n197 = invoke class="Tree" method="Edit Tree Items.Delete"(reference=w443, error in=w442, "tag"=w444, "Delete Children"=FALSE ("Delete Children?")) -> (reference out=w426:refnum<vi>, error out=w419:errorcluster)  [unwired: 1 in, 3 out]
            n198 = Build Array(w424) -> (w423:refnum<vi>[])
            n199 = Decrement(x=w422) -> (x-1=w428:i32)
            n200 = call "FormatTableStyle.vi"("Format Command"=FormatTableStyle_Commands."Uncolour Row", "Error In"=w419, "Row Index"=w422, "Table reference Array"=w423) -> ("Error Out"=w420:errorcluster)  [unwired: 7 in]
            n201 = call "FormatTree&TableStyle.vi"("Format Command"=FormatTree&TableStyle_Commands."Colour Row", "Error In"=w420, "Row Index"=w428, "Tbl Refnum"=w424, "Tree Refnum"=w426) -> ("Error Out"=w433:errorcluster)  [unwired: 6 in]
            n202 = property class="Tree"(reference=w426, error in=w433, "Active Item Row Number"=w428) -> (reference out=w431:refnum<vi>, error out=w432:errorcluster)
            n203 = call "Evaluate Macro_LOOPs.vi"("Error In"=w432, "Tree Refnum IN"=w431) -> ("Error Out"=w430:errorcluster, "Tree Refnum OUT"=w429:refnum<vi>)  [unwired: 7 in, 1 out]
            n204 = Close Reference(reference=w429, error in (no error)=w430) -> (error out=w427:errorcluster)
          }
        }
      }
      event Value Change {
        n205 = event-data() -> ()  [unwired: 1 in, 1 out]
        n206 = Unbundle By Name(w463) -> ("Created Macro"=w455:refnum<vi>)
        n207 = call "Tree_GetTag FromIndex.vi"("Error In"=w453, "Index IN"=w454, "Tree Refnum IN"=w455) -> ("Error Out"=w452:errorcluster, "Tag OUT"=w450:string, "Tree Refnum OUT"=w451:refnum<vi>)  [unwired: 6 in]
        n208 = call "Tree_GetTextFromTag.vi"("Error In"=w452, "Tag IN"=w450, "Tree Refnum IN"=w451) -> ("Error Out"=w458:errorcluster, "String OUT"=w456:string, "Tree Refnum OUT"=w457:refnum<vi>)  [unwired: 6 in]
        n209 = Close Reference(reference=w457, error in (no error)=w458) -> (error out=w459:errorcluster)
        n210 = case shown="\"Pause\"" w456 {
          tunnel: w459 -> [w483 w487 w491 w495 w499]
          tunnel: [w484 w488 w491 w494 w498] -> w464
          tunnel: [w482 w486 T9 {"Action"=enum."Unknown", "Arguments"=[]} ("Macro Commands") w492 w497] -> w461
          tunnel: [w481 w485 TRUE ("Cancelled?") w493 w496] -> w460
          frame "Pause" {
            n211 = call "Dialog_Enter Wait Duration.vi"("Error In"=w483) -> ("Error Out"=w484:errorcluster, "Cancelled?"=w481:bool, "Macro Commands"=w482:T9)  [unwired: 8 in]
          }
          frame "Load.Settings.File" {
            n212 = call "Dialog_Enter Load Setup File Path.vi"("Error In"=w487) -> ("Error Out"=w488:errorcluster, "Cancelled?"=w485:bool, "Macro Commands"=w486:T9)  [unwired: 8 in]
          }
          frame Default {
            # "Do nothing"
          }
          frame "Move.To.Position" {
            n213 = call "Dialog_Enter Stage Position.vi"("Error In"=w495) -> ("Error Out"=w494:errorcluster, "Cancelled?"=w493:bool, "Macro Commands"=w492:T9)  [unwired: 8 in]
          }
          frame "LOOP.Start" {
            n214 = call "Dialog_Enter Loop Iterations.vi"("Error In"=w499) -> ("Error Out"=w498:errorcluster, "Cancelled?"=w496:bool, "Macro Commands"=w497:T9)  [unwired: 8 in]
          }
        }
        n215 = case shown="False" w460 {
          tunnel: w464 -> [w473 w480]
          tunnel: w463 -> [w470 _]
          tunnel: [w468 w480] -> w462
          tunnel: w461 -> [w466 _]
          tunnel: w454 -> [w465 _]
          frame False {
            n216 = call "FGV_MacroGen.vi"("Final Index"=w465, "MacroFGV_Commands"=FGV_MacroGen_Commands."Edit Item", "Error In"=w473, "Macro Command IN"=w466) -> ("Error Out"=w472:errorcluster, "Macro Cluster Array"=w471:T9[])  [unwired: 5 in, 1 out]
            n217 = call "Macro Cluster to Text.vi"("Error In"=w472, "Macro Cluster Array IN"=w471) -> ("Error Out"=w475:errorcluster, "Argument List (Txt)"=w467:string[])  [unwired: 7 in, 1 out]
            n218 = Unbundle By Name(w470) -> ("Params Table"=w469:refnum<vi>)
            n219 = Build Array(w467) -> (w478:string[][])
            n220 = Transpose 2D Array(2D array=w478) -> (transposed array=w479:string[][])
            n221 = property class="Tbl (strict)"(reference=w469, error in=w475, "Value"=w479) -> (reference out=w477:refnum<vi>, error out=w476:errorcluster)
            n222 = Close Reference(reference=w477, error in (no error)=w476) -> (error out=w468:errorcluster)
          }
          frame True {
            # "Cancelled - Do Nothing!"
          }
        }
      }
      event "stop": Value Change {
        n223 = event-data() -> ()  [unwired: 1 in, 1 out]
      }
    }
    n224 = Unbundle(w22) -> ("status"=w20:bool)  [unwired: 2 out]
    n225 = Or(x=w20, y=w21) -> (x .or. y?=w19:bool)
  }
  n226 = call <vilib>:"Simple Error Handler.vi"("error in (no error)"=w16) -> ()  [unwired: 4 in, 5 out]
